vi "VI_principal.vi"() -> ()   [LabVIEW 2020]
uses:
  <vilib>/LabVIEW Open Source Project/Epoch Date & Time/epoch.UNIX/Epoch.UNIX.lvclass
panel:
  in  "Tab Control":enum32{"Fase A", "Fase B", "Fase C"}(tab)
  out "Potencia A 2":waveform(dbl)
  out "Potencia A":waveform(dbl)(graph)
  out "Potencia B 2":waveform(dbl)
  out "Potencia B":waveform(dbl)(graph)
  out "Potencia C 2":waveform(dbl)
  out "Potencia C":waveform(dbl)(graph)
  in  "stop":bool
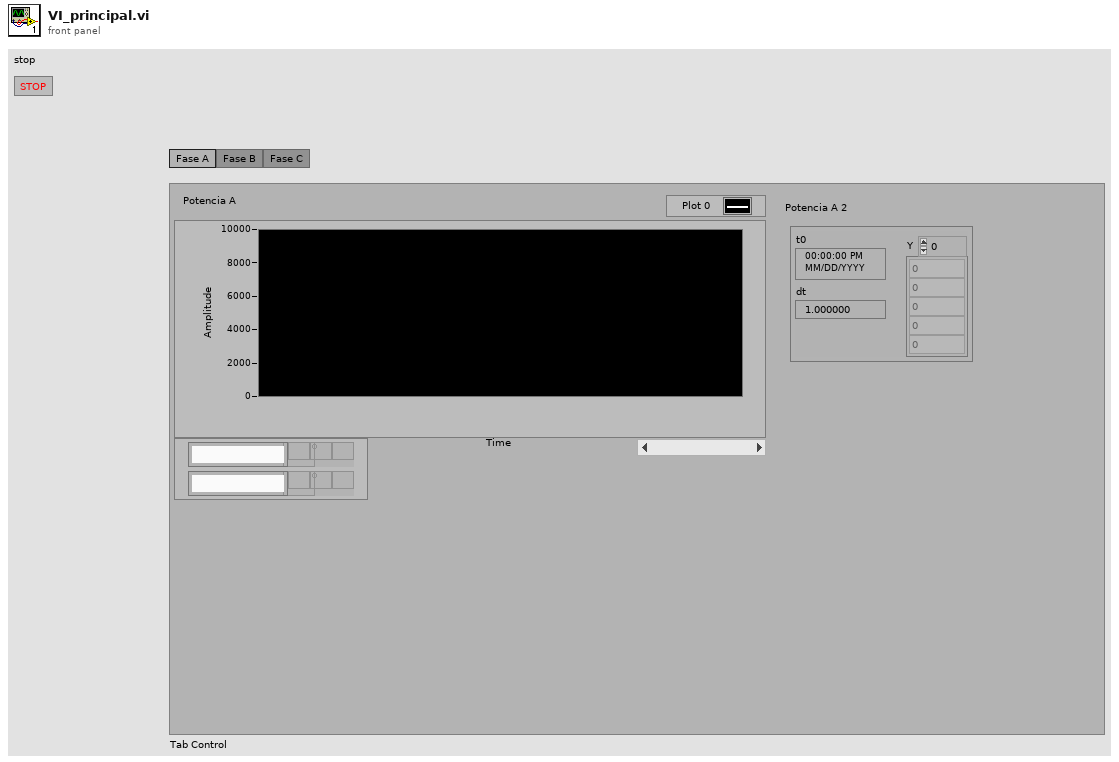
[diagram p1: front panel]
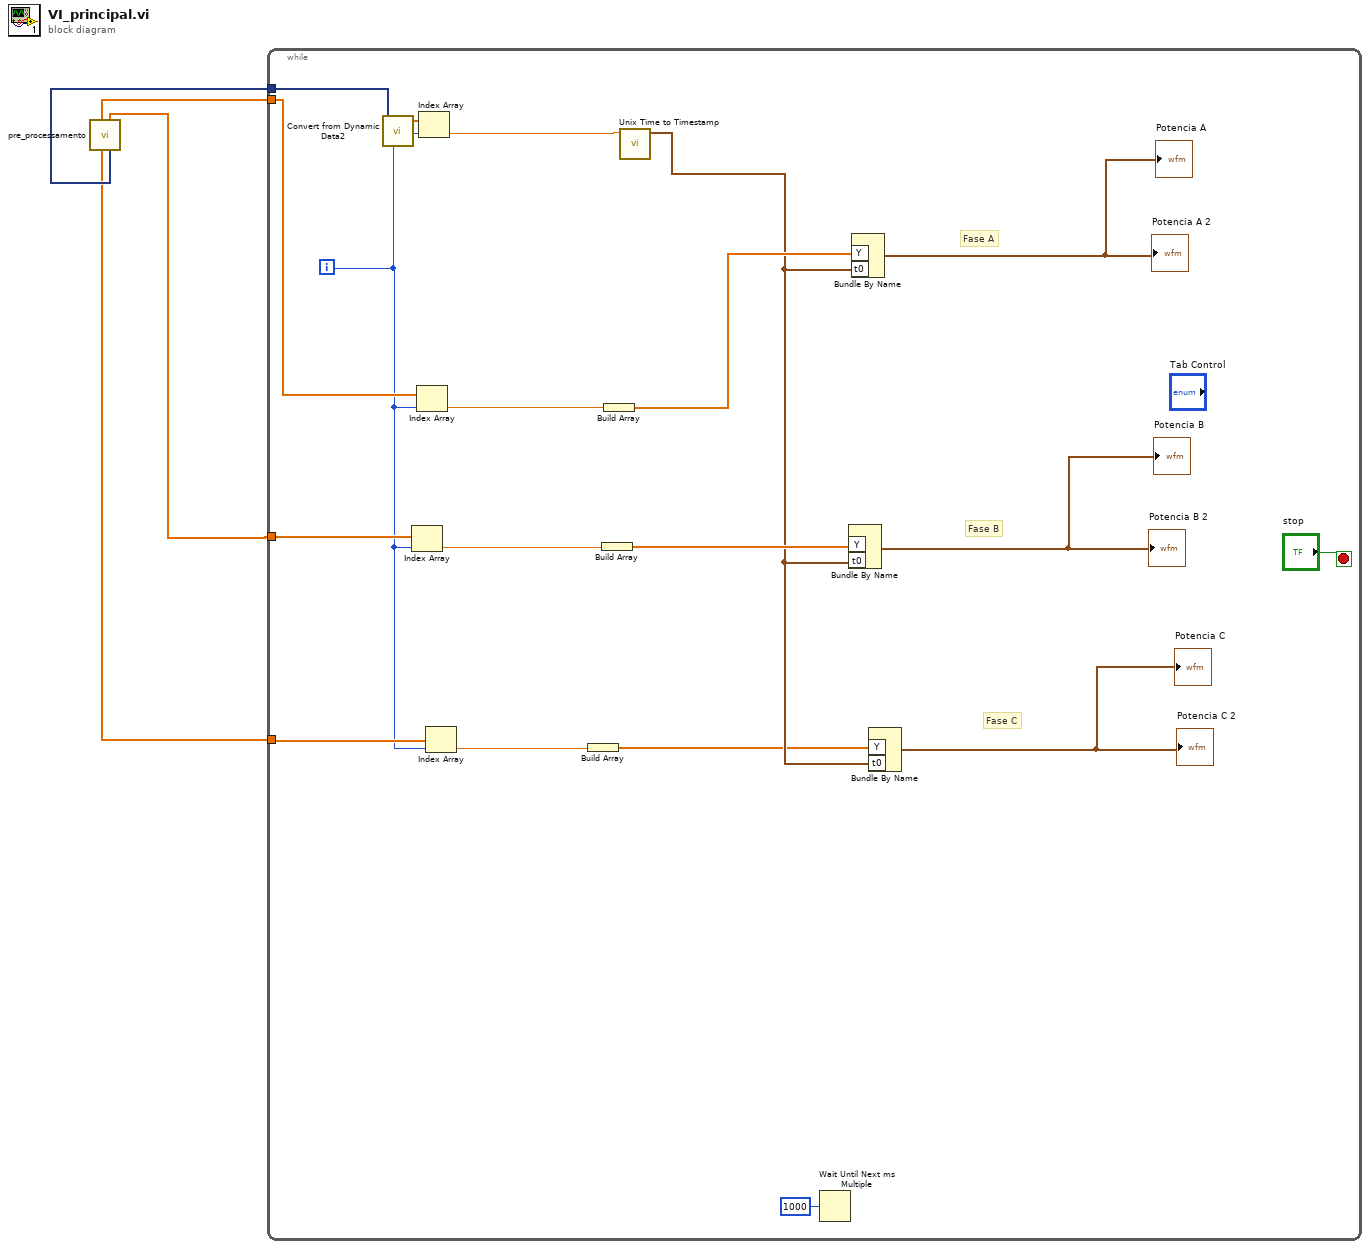
[diagram p0: block diagram]
diagram:
  n1 = call "pre_processamento.vi"() -> ("TimeStamp"=w3:dynamicdata, "Potencia B"=w2:dbl[], "Potencia C"=w1:dbl[], "Potencia A"=w4:dbl[])  [unwired: 2 in, 6 out]
  n2 = while {
    tunnel: w4 -> [w16]
    tunnel: w3 -> [w23]
    tunnel: w2 -> [w14]
    tunnel: w1 -> [w10]
    i -> [w9]
    stop <- "stop" stop-if-true
    # "Fase C"
    # "Fase B"
    # "Fase A"
    n3 = call "Convert from Dynamic Data2"("Dynamic Data Type"=w23) -> ("Array"=w17:dbl[])  [unwired: 3 in]
    n4 = Index Array(array=w14, index=w9) -> (element=w13:dbl)
    n5 = Index Array(array=w16, index=w9) -> (element=w21:dbl)
    n6 = Index Array(array=w17, index=w9) -> (element=w22:dbl)
    n7 = Index Array(array=w10, index=w9) -> (element=w8:dbl)
    n8 = Build Array(w8) -> (w6:dbl[])
    n9 = Build Array(w13) -> (w12:dbl[])
    n10 = Build Array(w21) -> (w15:dbl[])
    n11 = call <vilib>:"Unix Time to Timestamp.vi"("Unix Time (s)"=w22) -> ("Timestamp"=w7:timestamp)  [unwired: 9 in, 1 out]
    n12 = Wait Until Next ms Multiple(millisecond multiple=u32 1000) -> ()  [unwired: 1 out]
    n13 = Bundle By Name("Y"=w12, "t0"=w7) -> (→"Potencia B 2" →"Potencia B":waveform(dbl))  [unwired: 1 in]
    n14 = Bundle By Name("Y"=w15, "t0"=w7) -> (→"Potencia A 2" →"Potencia A":waveform(dbl))  [unwired: 1 in]
    n15 = Bundle By Name("Y"=w6, "t0"=w7) -> (→"Potencia C 2" →"Potencia C":waveform(dbl))  [unwired: 1 in]
  }
